vi "Set Waveform Factory.vi"(10 "WaveformFactory":refnum<class "Waveform Factory.lvclass">, 11 "Model in":refnum<class "Model.lvclass">) -> (3 "Model out":refnum<class "Model.lvclass">)   [LabVIEW 2016]
uses:
  Model.lvclass
  Waveforms/Waveform Factory/Waveform Factory.lvclass
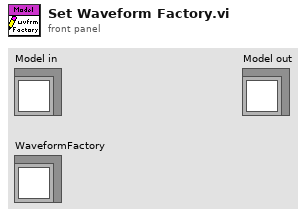
[diagram p1: front panel]
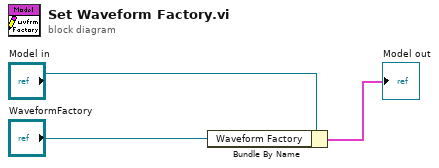
[diagram p0: block diagram]
diagram:
  n1 = Bundle By Name(cluster="Model in", "Waveform Factory"="WaveformFactory") -> (→"Model out":cluster{})
